vi "voltageAverage.vi"(0 "waveform":waveform(dbl)) -> (1 "avgVoltage":dbl, 2 "numSamplesAvg":i32)   [LabVIEW 2018]
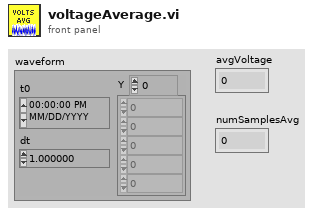
[diagram p1: front panel]
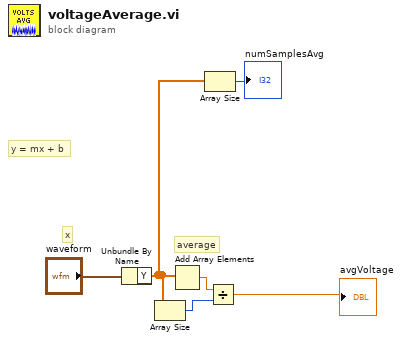
[diagram p0: block diagram]
diagram:
  # "x"
  # "y = mx + b"
  # "average"
  n1 = Unbundle By Name("waveform") -> ("Y"=w1:dbl[])
  n2 = Array Size(array=w1) -> (size(s)=w5:i32)
  n3 = Add Array Elements(numeric array=w1) -> (sum=w6:dbl)
  n4 = Array Size(array=w1) -> (size(s)=→"numSamplesAvg":i32)
  n5 = Divide(x=w6, y=w5) -> (x/y=→"avgVoltage":dbl)
